vi "finalize initialization.vi"(8 "error in":errorcluster, 10 "configuration in":refnum<class "fixed channel configuration.lvclass">, 11 "System Diagnostics runtime in":refnum<class "System Diagnostics runtime.lvclass">) -> (0 "error out":errorcluster, 3 "System Diagnostics runtime out":refnum<class "System Diagnostics runtime.lvclass">)   [LabVIEW 2013, in "System Diagnostics runtime.lvclass"]
uses:
  System Diagnostics runtime.lvclass
  <vilib>/NI/Tag Bus Data Framework/fixed module parent/module/configuration/fixed channel configuration.lvclass
  configuration/System Diagnostics configuration.lvclass
  System Diagnostics runtime.lvclass/System Diagnostics runtime.ctl
  <vilib>/nisyscfg/nisyscfg.lvlib
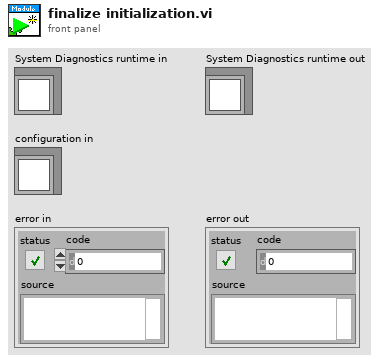
[diagram p1: front panel]
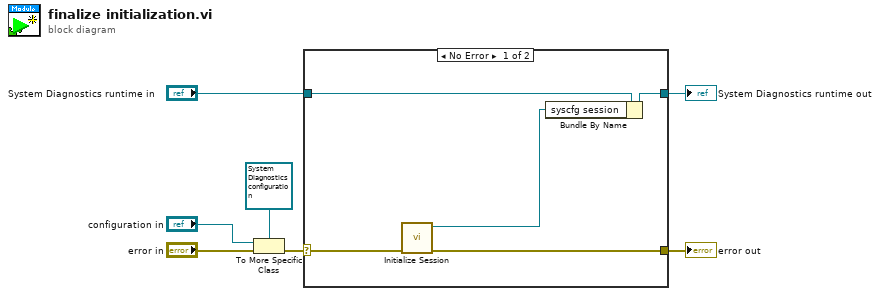
[diagram p0: block diagram]
diagram:
  n1 = To More Specific Class(target class=refnum<class "System Diagnostics configuration.lvclass"> refnum ("user module configuration"), reference="configuration in", error in="error in") -> (error out=w4:errorcluster)  [unwired: 1 out]
  n2 = case shown="No Error" w4 {
    selector: w4 -> [w10 w13]
    tunnel: [w11 w14] -> w3
    tunnel: "System Diagnostics runtime in" -> [w12 w14]
    tunnel: [w9 w13] -> w1
    frame No Error {
      n3 = call <vilib>:"Initialize Session.vi"("error in (no error)"=w10) -> ("error out"=w9:errorcluster, "Session out"=w8:refnum<k21>)  [unwired: 9 in]
      n4 = Bundle By Name(cluster=w12, "syscfg session"=w8) -> (w11:refnum<class "System Diagnostics runtime.lvclass">)
    }
    frame Error {
    }
  }
  "error out" <- w1
  "System Diagnostics runtime out" <- w3
